vi "LockinDAQ.Create.AI.vi"(8 "error in (no error)":errorcluster, 11 "LockinDAQ":refnum<class "LockinDAQ.lvclass">) -> (0 "error out":errorcluster, 3 "LockinDAQ out":refnum<class "LockinDAQ.lvclass">)   [LabVIEW 2016, in "LockinDAQ.lvclass"]
uses:
  LockinDAQ.lvclass
  LockinDAQ.lvclass/LockinDAQ.ctl
  <vilib>/DAQmx/create/channels.llb/DAQmx Create Channel (AI-Voltage-Basic).vi
  <resource>/objmgr/daqmx.rc
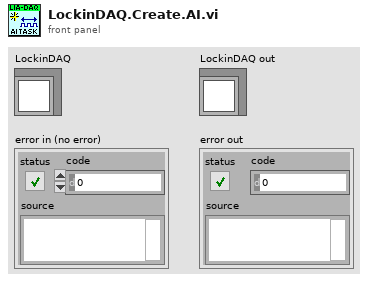
[diagram p1: front panel]
types:
  T1 = typedef "LockinDAQ.lvclass/AI.config-array.ctl" = T2[]
  T2 = typedef "LockinDAQ.lvclass/AI.config-cluster.ctl" = cluster{"AI.channels":tag, "AI.Coupling":T3, "AI.Range":T4, "input terminal configuration":i32, "DAQ Type":T5}
  T3 = typedef "LockinDAQ.lvclass/AI.coupling-enum.ctl" = u16
  T4 = typedef "LockinDAQ.lvclass/446xAI-enum.ctl" = enum16{"±0.316 V", "±1.00 V", "±3.16 V", "±10.0 V", "±31.6 V", "±42.4 V"}
  T5 = typedef "LockinDAQ.lvclass/DAQType-enum.ctl" = enum16{"None", "USB 4431", "PXI 446x"}
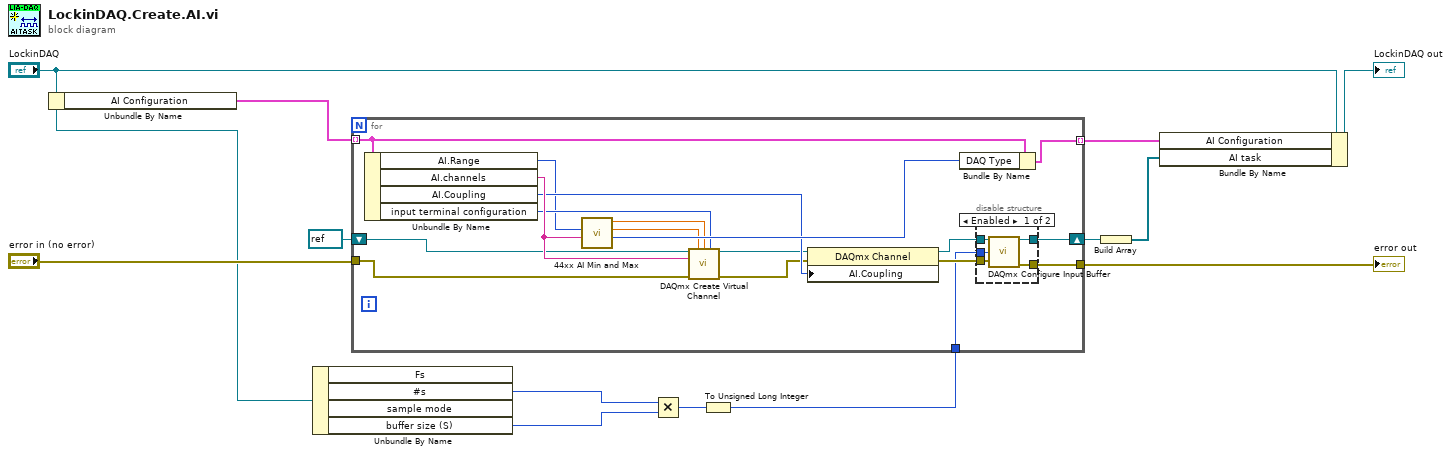
[diagram p0: block diagram]
diagram:
  n1 = Unbundle By Name("LockinDAQ") -> ("AI Configuration"=w10:T1)
  n2 = Unbundle By Name("LockinDAQ") -> ("#s"=w8:i32, "buffer size (S)"=w7:u32)  [unwired: 2 out]
  n3 = Multiply(x=w8, y=w7) -> (x*y=w9:u32)
  n4 = To Unsigned Long Integer(number=w9) -> (unsigned 32bit integer=w6:u32)
  n5 = for {
    tunnel: [w16] -> w4 mode=indexing
    tunnel: w10 -> [w21] mode=indexing
    tunnel: "error in (no error)" -> [w22]
    tunnel: [w19] -> w12
    tunnel: w6 -> [w17]
    shift-right: [w15] -> w3
    shift-left: refnum<k21> refnum ("task out") -> [w14]
    n6 = Unbundle By Name(w21) -> ("AI.Range"=w27:T4, "AI.channels"=w31:tag, "AI.Coupling"=w28:T3, "input terminal configuration"=w29:i32)
    n7 = call "44xx AI Min and Max.vi"("AI.channels"=w31, "446x AI"=w27) -> ("DAQ Type"=w30:T5, "AI.Max"=w25:dbl, "AI.Min"=w26:dbl)  [unwired: 7 in]
    n8 = call-poly <vilib>:"DAQmx Create Virtual Channel.vi"("task in"=w14, "maximum value"=w25, "minimum value"=w26, "input terminal configuration"=w29, "physical channels"=w31, "error in"=w22) -> ("task out"=w23:refnum<k21>, "error out"=w24:errorcluster)  [unwired: 8 in]
    n9 = property class="DAQmx Channel"(reference=w23, error in=w24, "AI.Coupling"=w28) -> (reference out=w18:refnum<k21>, error out=w20:errorcluster)
    n10 = Bundle By Name(cluster=w21, "DAQ Type"=w30) -> (w16:T2)
    n11 = disable-structure shown="Enabled" {
      disable-tunnel: w20 -> [w36 w37]
      disable-tunnel: [w35 w37] -> w19
      disable-tunnel: w18 -> [w34 w38]
      disable-tunnel: w17 -> [w33 _]
      disable-tunnel: [w32 w38] -> w15
      frame Enabled {
        n12 = call <vilib>:"DAQmx Configure Input Buffer.vi"("task/channels in"=w34, "buffer size (in samples per channel)"=w33, "error in"=w36) -> ("task out"=w32:refnum<k21>, "error out"=w35:errorcluster)  [unwired: 11 in]
      }
      frame Disabled {
      }
    }
  }
  "error out" <- w12
  n13 = Build Array(w3) -> (w2:refnum<k21>[])
  n14 = Bundle By Name(cluster="LockinDAQ", "AI Configuration"=w4, "AI task"=w2) -> (→"LockinDAQ out":refnum<class "LockinDAQ.lvclass">)
